vi "Untitled 3 (SubVI).vi"(4 "sequence result header":string[](array[string]), 6 "std seq number":i32, 7 "unknown cycle":string[](array[string]), 9 "Cycle data by seq":dbl[][][](array[numeric]), 11 "cycle results dbl":dbl[](array[numeric])) -> (1 "output array":dbl[](array[numeric]))   [LabVIEW 2016]
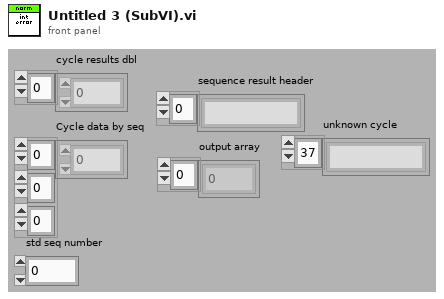
[diagram p1: front panel]
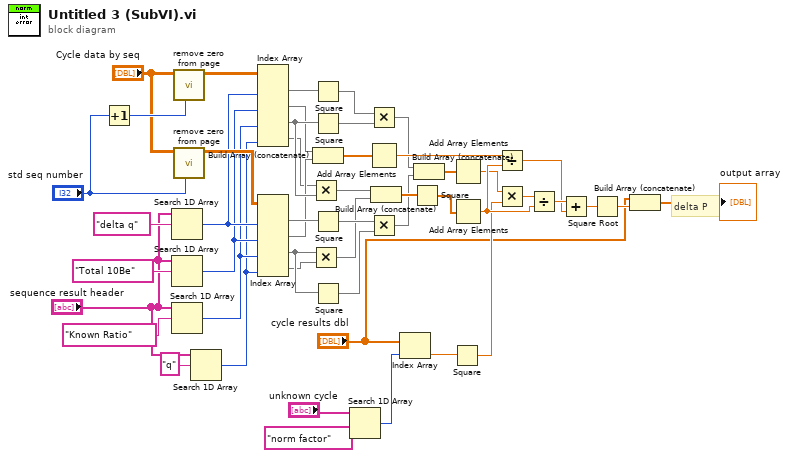
[diagram p0: block diagram]
diagram:
  # "delta P"
  n1 = Increment(x="std seq number") -> (x+1=w16:i32)
  n2 = Search 1D Array(1D array="sequence result header", element="delta q") -> (index of element=w7:i32)  [unwired: 1 in]
  n3 = Search 1D Array(1D array="sequence result header", element="Total 10Be") -> (index of element=w6:i32)  [unwired: 1 in]
  n4 = Search 1D Array(1D array="sequence result header", element="Known Ratio") -> (index of element=w5:i32)  [unwired: 1 in]
  n5 = call "remove zero from page.vi"("page number"=w16, "Cycle data by seq"="Cycle data by seq") -> ("array w/ subset deleted"=w17:dbl[][])  [unwired: 9 in]
  n6 = call "remove zero from page.vi"("page number"="std seq number", "Cycle data by seq"="Cycle data by seq") -> ("array w/ subset deleted"=w18:dbl[][])  [unwired: 9 in]
  n7 = Search 1D Array(1D array="sequence result header", element="q") -> (index of element=w4:i32)  [unwired: 1 in]
  n8 = Index Array(array=w17, index (col) #1=w7, index (col) #2=w6, index (col) #3=w5, index (col) #4=w4) -> (element #1=w28:dbl[], element #2=w23:dbl[], element #3=w30:dbl[], element #4=w20:dbl[])  [unwired: 4 in]
  n9 = Index Array(array=w18, index (col) #1=w7, index (col) #2=w6, index (col) #3=w5, index (col) #4=w4) -> (element #1=w32:dbl[], element #2=w24:dbl[], element #3=w34:dbl[], element #4=w19:dbl[])  [unwired: 4 in]
  n10 = Multiply(x=w20, y=w30) -> (x*y=w22:dbl[])
  n11 = Multiply(x=w34, y=w19) -> (x*y=w21:dbl[])
  n12 = Square(x=w28) -> (x^2=w29:dbl[])
  n13 = Square(x=w30) -> (x^2=w31:dbl[])
  n14 = Build Array (concatenate)(w23, w24) -> (w42:dbl[])
  n15 = Square(x=w32) -> (x^2=w33:dbl[])
  n16 = Square(x=w34) -> (x^2=w35:dbl[])
  n17 = Search 1D Array(1D array="unknown cycle", element="norm factor") -> (index of element=w1:i32)  [unwired: 1 in]
  n18 = Multiply(x=w29, y=w31) -> (x*y=w26:dbl[])
  n19 = Add Array Elements(numeric array=w42) -> (sum=w43:dbl)
  n20 = Multiply(x=w33, y=w35) -> (x*y=w27:dbl[])
  n21 = Build Array (concatenate)(w22, w21) -> (w36:dbl[])
  n22 = Index Array(array="cycle results dbl", index=w1) -> (element=w37:dbl)
  n23 = Square(x=w36) -> (x^2=w41:dbl[])
  n24 = Build Array (concatenate)(w26, w27) -> (w39:dbl[])
  n25 = Square(x=w37) -> (x^2=w44:dbl)
  n26 = Add Array Elements(numeric array=w39) -> (sum=w40:dbl)
  n27 = Add Array Elements(numeric array=w41) -> (sum=w45:dbl)
  n28 = Divide(x=w43, y=w45) -> (x/y=w38:dbl)
  n29 = Multiply(x=w40, y=w44) -> (x*y=w46:dbl)
  n30 = Divide(x=w46, y=w45) -> (x/y=w47:dbl)
  n31 = Add(x=w47, y=w38) -> (x+y=w48:dbl)
  n32 = Square Root(x=w48) -> (sqrt(x)=w49:dbl)
  n33 = Build Array (concatenate)("cycle results dbl", w49) -> (→"output array":dbl[])
